vi "Add ClassLib to Project.vi"() -> ()   [LabVIEW 2019, in "VI Scripting Tools.lvlib"]
uses:
  Source/VI Scripting Tools/Library/VI Scripting Tools.lvlib
panel:
  out "error out":errorcluster
  out "New Library Path":path
  out "Build Specification Names":string[](array[string])
  in  "error in (no error)":errorcluster
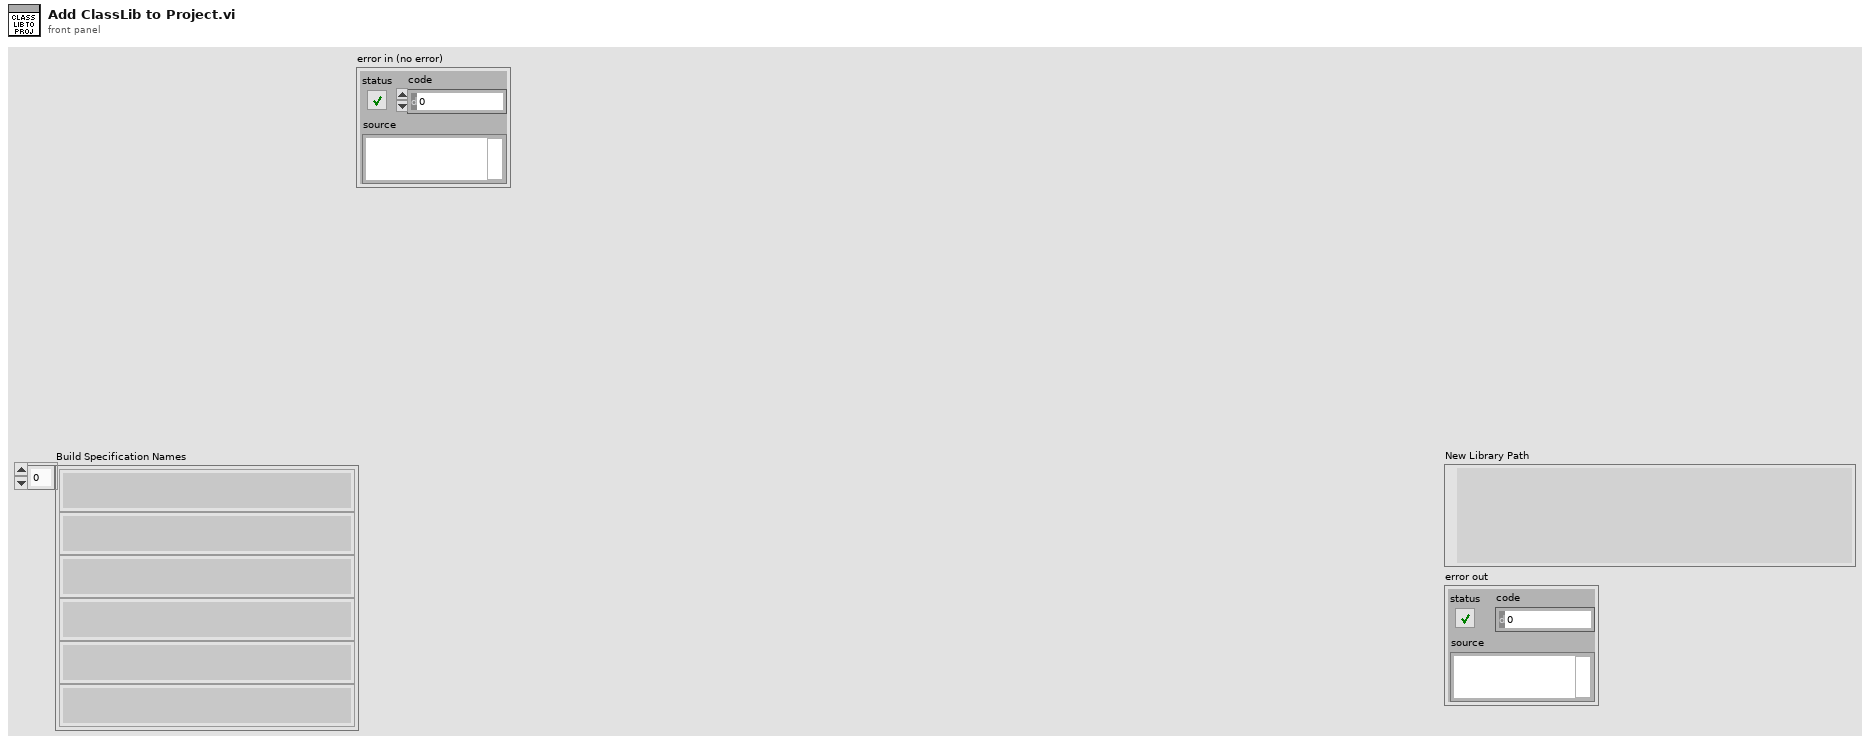
[diagram p1: front panel]
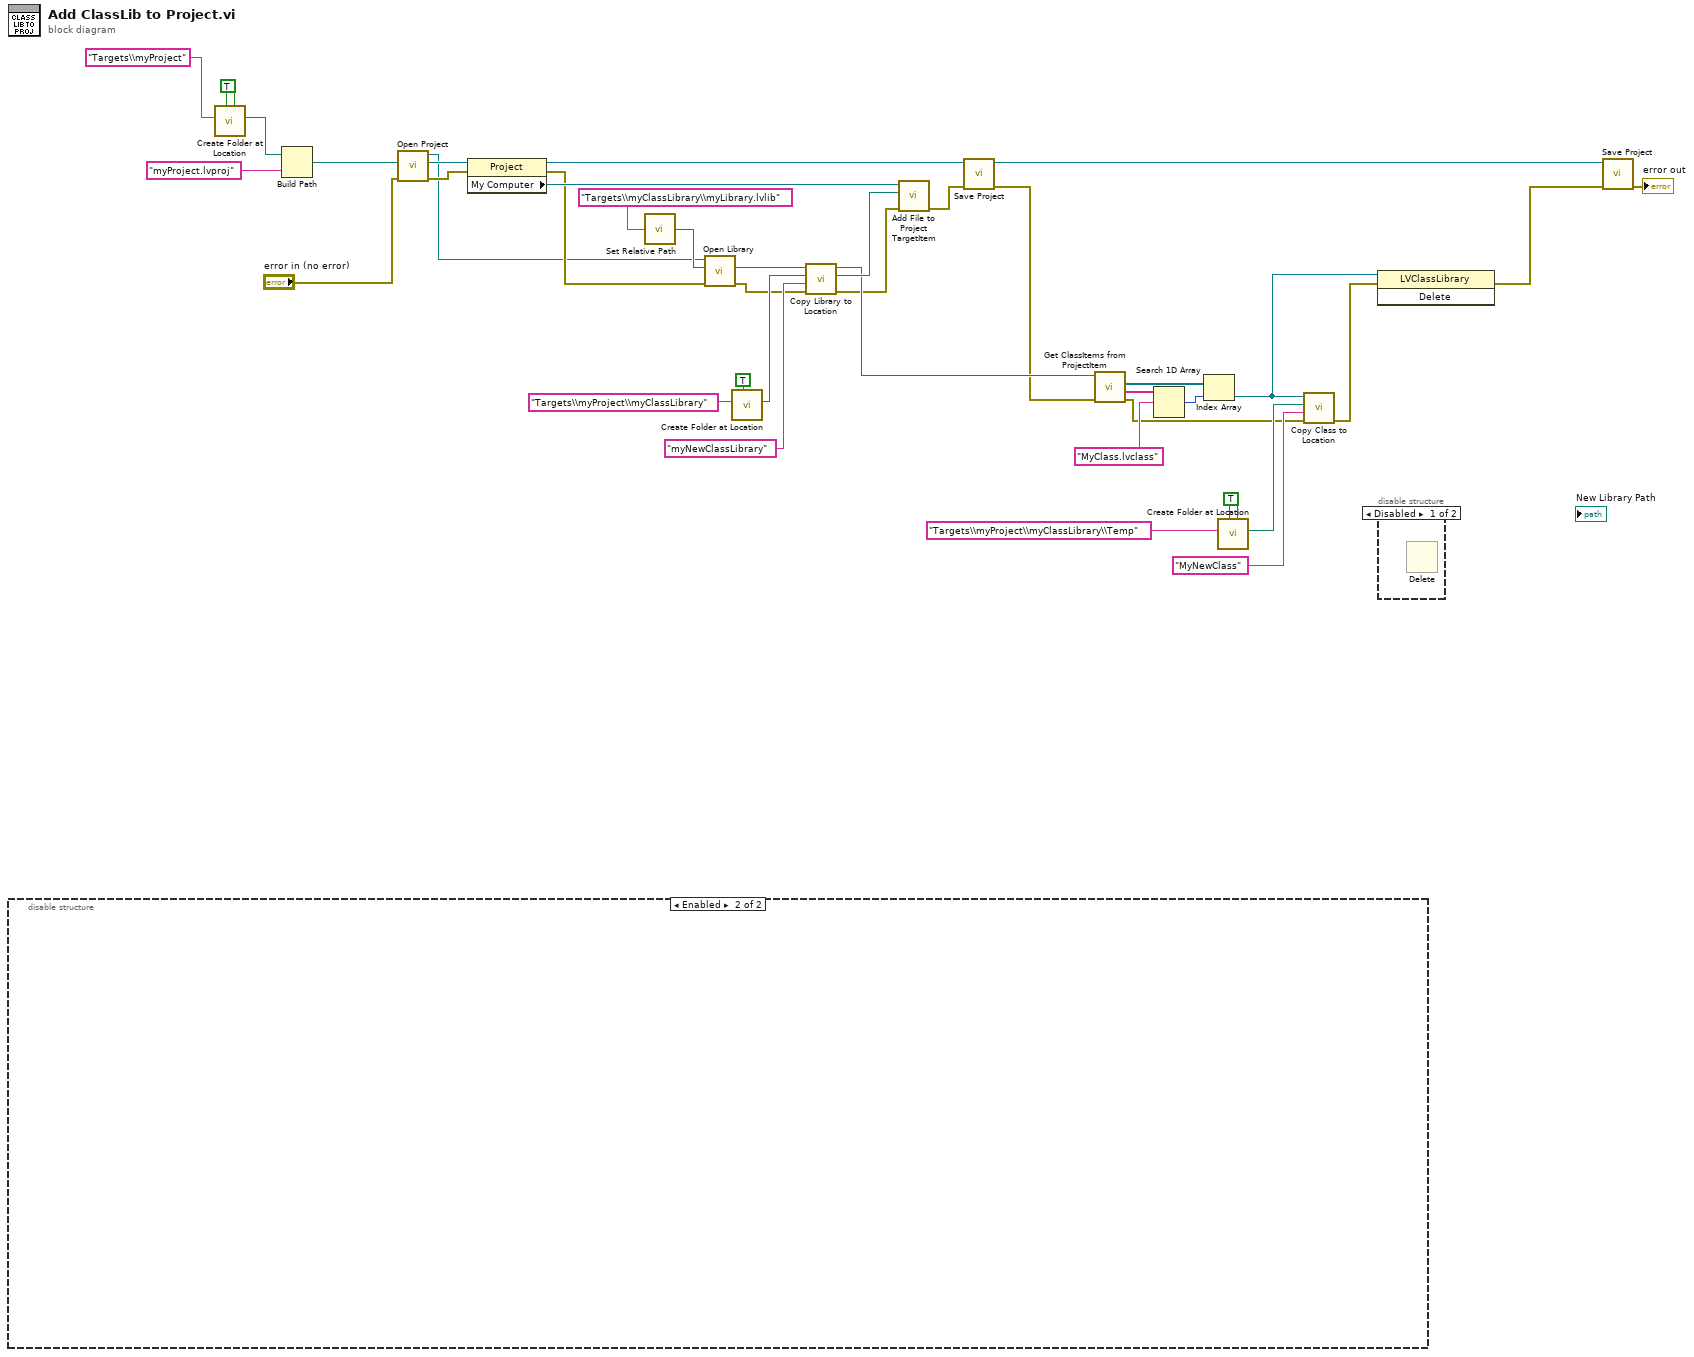
[diagram p0: block diagram]
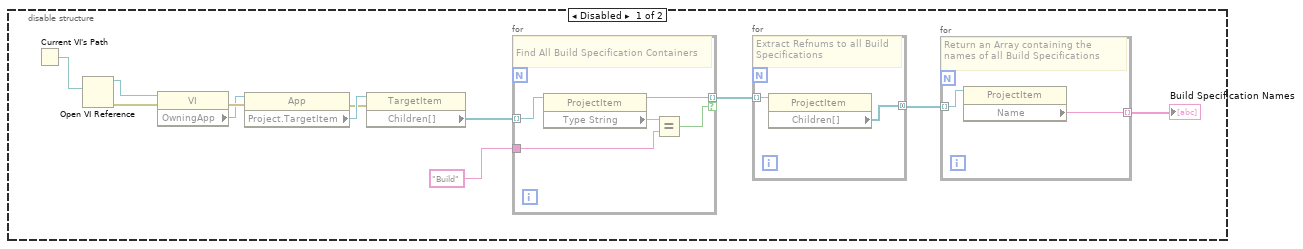
[diagram p3: hidden frame]
diagram:
  w16 = TRUE ("Use Relative")
  w38 = TRUE ("Use Relative")
  n1 = disable-structure shown="Enabled" {
    frame Disabled {
      n2 = Current VI's Path() -> (path=w42:path)
      n3 = Open VI Reference(vi path=w42) -> (vi reference=w43:refnum<vi>, error out=w44:errorcluster)  [unwired: 5 in]
      n4 = property class="VI"(reference=w43, error in=w44) -> (error out=w50:errorcluster, "OwningApp"=w45:refnum<vi>)  [unwired: 1 out]
      n5 = property class="App"(reference=w45, error in=w50) -> (error out=w46:errorcluster, "Project.TargetItem"=w47:refnum<vi>)  [unwired: 1 out]
      n6 = property class="TargetItem"(reference=w47, error in=w46) -> ("Children[]"=w48:refnum<vi>[])  [unwired: 2 out]
      n7 = for {
        tunnel: w48 -> [w60] mode=indexing
        tunnel: [w58] -> w49 mode=indexing if=w57
        tunnel: "Build" ("y") -> [w56]
        # "Find All Build Specification Containers"
        n8 = property class="ProjectItem"(reference=w60) -> (reference out=w58:refnum<vi>, "Type String"=w59:string)  [unwired: 1 in, 1 out]
        n9 = Equal?(x=w59, y=w56) -> (x = y?=w57:bool)
      }
      n10 = for {
        tunnel: w49 -> [w55] mode=indexing
        tunnel: [w54] -> w40 mode=concatenating
        # "Extract Refnums to all Build Specifications"
        n11 = property class="ProjectItem"(reference=w55) -> ("Children[]"=w54:refnum<vi>[])  [unwired: 1 in, 2 out]
      }
      n12 = for {
        tunnel: w40 -> [w53] mode=indexing
        tunnel: [w52] -> w41 mode=indexing
        # "Return an Array containing the names of all Build Specifications"
        n13 = property class="ProjectItem"(reference=w53) -> ("Name"=w52:string)  [unwired: 1 in, 2 out]
      }
      "Build Specification Names" <- w41
    }
    frame Enabled {
    }
  }
  n14 = call "Create Folder at Location.vi"("Override existing"=w38, "Use Relative"=w38, "Path"="Targets\\myProject") -> ("Full path out"=w30:path)  [unwired: 7 in, 1 out]
  n15 = Build Path(base path=w30, name or relative path="myProject.lvproj") -> (appended path=w37:path)
  n16 = call "Open Project.vi"("error in (no error)"="error in (no error)", "Project Path in"=w37) -> ("error out"=w31:errorcluster, "Project out"=w34:refnum<vi>, "Application reference out"=w21:refnum<vi>)  [unwired: 7 in]
  n17 = property class="Project"(reference=w34, error in=w31) -> (reference out=w9:refnum<vi>, error out=w25:errorcluster, "My Computer"=w33:refnum<vi>)
  n18 = call "Set Relative Path.vi"("App Relative Path"="Targets\\myClassLibrary\\myLibrary.lvlib") -> ("Full Path"=w24:path)
  n19 = call "Open Library.vi"("error in (no error)"=w25, "Full Path"=w24, "Application reference in"=w21) -> ("error out"=w23:errorcluster, "Library out"=w22:refnum<vi>)  [unwired: 6 in, 1 out]
  n20 = call "Create Folder at Location.vi"("Use Relative"=TRUE, "Path"="Targets\\myProject\\myClassLibrary") -> ("Full path out"=w27:path)  [unwired: 8 in, 1 out]
  n21 = call "Copy Library to Location.vi"("error in (no error)"=w23, "Copy Name"="myNewClassLibrary" ("name or relative path"), "Copy location"=w27, "Library in"=w22) -> ("error out"=w10:errorcluster, "New Lib Path"=w12:path, "Library out"=w11:refnum<vi>)  [unwired: 5 in]
  n22 = call "Add File to Project TargetItem.vi"("error in (no error)"=w10, "New File Location"=w12, "Project TargetItem in"=w33) -> ("error out"=w8:errorcluster)  [unwired: 6 in, 2 out]
  n23 = call "Save Project.vi"("error in (no error)"=w8, "Project in"=w9) -> ("error out"=w7:errorcluster, "Project out"=w6:refnum<vi>)  [unwired: 8 in]
  n24 = call "Get ClassItems from ProjectItem.vi"("error in (no error)"=w7, "ProjectItem in"=w11) -> ("error out"=w2:errorcluster, "Class Item Names"=w20:string[], "Class Items"=w18:refnum<vi>[])  [unwired: 6 in, 1 out]
  n25 = Search 1D Array(1D array=w20, element="MyClass.lvclass") -> (index of element=w17:i32)  [unwired: 1 in]
  n26 = Index Array(array=w18, index=w17) -> (element=w1:refnum<vi>)
  n27 = call "Create Folder at Location.vi"("Override existing"=w16, "Use Relative"=w16, "Path"="Targets\\myProject\\myClassLibrary\\Temp") -> ("Full path out"=w15:path)  [unwired: 7 in, 1 out]
  n28 = call "Copy Class to Location.vi"("error in (no error)"=w2, "New Name"="MyNewClass", "Full path in"=w15, "LVClassLibrary in"=w1) -> ("error out"=w3:errorcluster)  [unwired: 5 in, 2 out]
  n29 = invoke class="LVClassLibrary" method="Delete"(reference=w1, error in=w3) -> (error out=w4:errorcluster)  [unwired: 1 in, 2 out]
  n30 = disable-structure shown="Disabled" {
    frame Disabled {
      n31 = Delete() -> ()  [unwired: 5 in, 3 out]
    }
    frame Enabled {
    }
  }
  n32 = call "Save Project.vi"("error in (no error)"=w4, "Project in"=w6) -> ("error out"=→"error out":errorcluster)  [unwired: 8 in, 1 out]
